vi "DB-exe与fetch.vi"(8 "查询条件集":string[](array[string]), 11 "数据库引用":T1) -> ()   [LabVIEW 2013]
uses:
  <vilib>/addons/database/Connection.llb/Conn ObjectReference.ctl
  <vilib>/addons/database/Connection.llb/Conn Execute.vi
  <vilib>/addons/database/Recordset.llb/Rec Fetch Recordset Data (R).vi
  <vilib>/addons/database/Recordset.llb/Rec Destroy - Connection.vi
  <vilib>/addons/database/NI_Database_API.lvlib
panel:
  out "读取数据":variant[][](array[variant])
  in  "数据库BUSY标志引用":refnum<vi>
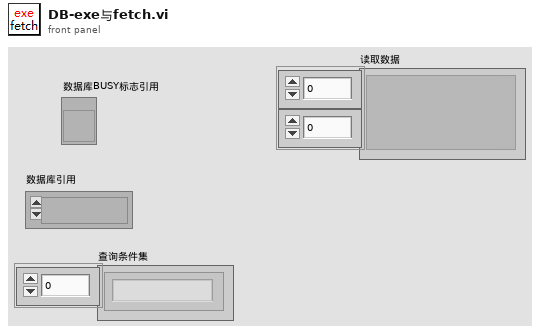
[diagram p1: front panel]
types:
  T1 = typedef "NI_Database_API.lvlib/Conn ObjectReference.ctl" = refnum<k1>
  T2 = typedef "NI_Database_API.lvlib/Rec ObjectReference.ctl" = refnum<k1>
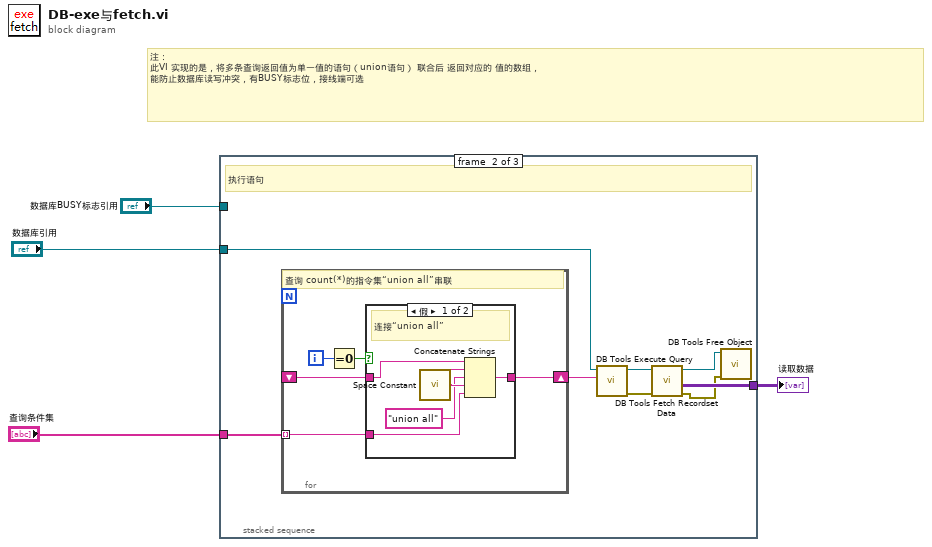
[diagram p0: block diagram]
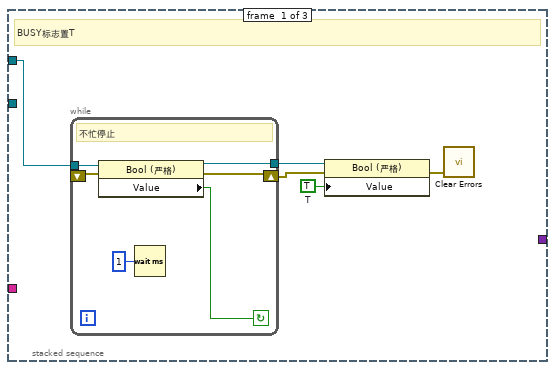
[diagram p2: hidden frame]
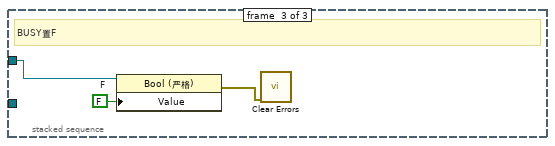
[diagram p4: hidden frame]
diagram:
  # "注：\n此VI 实现的是，将多条查询返回值为单一值的语句（union语句） 联合后 返回对应的 值的数组，\n能防止数据库读写冲突，有BUSY标志位，接线端可选"
  n1 = stacked-sequence {
    tunnel: "数据库引用" -> [_ w23 _]
    tunnel: "查询条件集" -> [_ w20 _]
    tunnel: "数据库BUSY标志引用" -> [w9 _ w37]
    tunnel: [_ w18 _] -> w1
    frame #0 {
      w7 = TRUE  # T
      # "BUSY标志置T"
      n2 = while {
        tunnel: w9 -> [w14]
        tunnel: [w12] -> w8
        shift-right: [w10] -> w6
        shift-left: _ -> [w11]
        stop <- w13 continue-if-true
        # "不忙停止"
        n3 = property class="Bool (严格)"(reference=w14, error in=w11) -> (reference out=w12:refnum<vi>, error out=w10:errorcluster, "Value"=w13:bool)
        n4 = Wait (ms)(milliseconds to wait=u32 1 ("等待时间（毫秒）")) -> ()  [unwired: 1 out]
      }
      n5 = property class="Bool (严格)"(reference=w8, error in=w6, "Value"=w7) -> (error out=w5:errorcluster)  [unwired: 1 out]
      n6 = call <vilib>:"Clear Errors.vi"("error in (no error)"=w5) -> ()  [unwired: 6 in, 1 out]
    }
    frame #1 {
      # "执行语句"
      n7 = for {
        tunnel: w20 -> [w26] mode=indexing
        shift-right: [w25] -> w19
        shift-left: _ -> [w24]
        i -> [w28]
        # "查询 count(*)的指令集“union all”串联"
        n8 = Equal To 0?(x=w28) -> (x = 0?=w27:bool)
        n9 = case shown="假" w27 {
          tunnel: w26 -> [w33 w34]
          tunnel: [w30 w34] -> w25
          tunnel: w24 -> [w29 _]
          frame False {
            # "连接“union all”"
            n10 = call <vilib>:"Space Constant.vi"() -> ("String"=w32:string)
            n11 = Concatenate Strings(w29, w32, "union all", w32, w33) -> (w30:string)
          }
          frame True {
            # "首次，不连接union"
          }
        }
      }
      n12 = call-poly <vilib>:"DB Tools Execute Query.vi"("SQL query"=w19, "connection reference"=w23) -> ("error out"=w22:errorcluster, "recordset reference"=w21:T2)  [unwired: 6 in]
      n13 = call-poly <vilib>:"DB Tools Fetch Recordset Data.vi"("error in (no error)"=w22, "recordset reference"=w21) -> ("error out"=w16:errorcluster, "recordset data"=w18:variant[][], "recordset reference out"=w17:T2)  [unwired: 3 in]
      n14 = call-poly <vilib>:"DB Tools Free Object.vi"("error in (no error)"=w16, "recordset reference"=w17) -> ()  [unwired: 8 in, 2 out]
    }
    frame #2 {
      w36 = FALSE  # F
      # "BUSY置F"
      n15 = property class="Bool (严格)"(reference=w37, "Value"=w36) -> (error out=w35:errorcluster)  [unwired: 1 in, 1 out]
      n16 = call <vilib>:"Clear Errors.vi"("error in (no error)"=w35) -> ()  [unwired: 6 in, 1 out]
    }
  }
  "读取数据" <- w1
